vi "create SimpleCredit.vi"(4 "Interest Rate Interval (s)":u32, 5 "Credit Limit Interval (s)":u32, 6 "Interest Rate":dbl, 7 "Credit Limit":dbl, 8 "error in (no error)":errorcluster, 9 "Initial Balance":dbl, 10 "Account Number":string, 11 "SimpleCredit in":refnum<class "SimpleCredit.lvclass">) -> (0 "error out":errorcluster, 3 "SimpleCredit out":refnum<class "SimpleCredit.lvclass">)   [LabVIEW 2020, in "SimpleCredit.lvclass"]
uses:
  SimpleCredit.lvclass
  C:/projects/budget_LabVIEW/Main Codeline/Software/Code/shared/AAccount/AAccount.lvclass
  C:/projects/budget_LabVIEW/Main Codeline/Software/Code/shared/ACreditAccount/ACreditAccount.lvclass
  C:/projects/budget_LabVIEW/Main Codeline/Software/Code/shared/AInterestAccount/AInterestAccount.lvclass
  SimpleCredit.lvclass/SimpleCredit.ctl
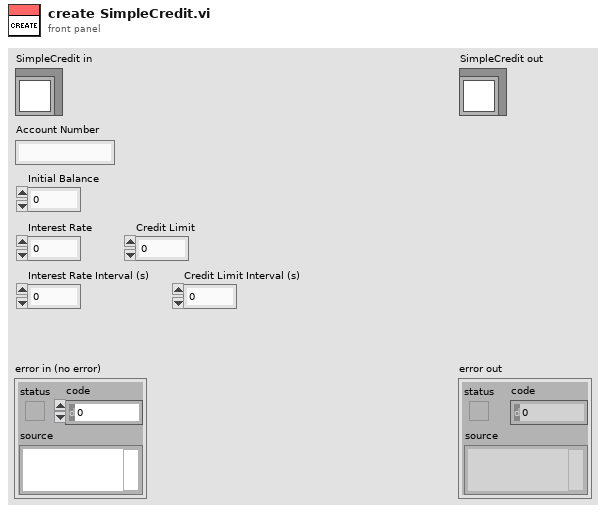
[diagram p1: front panel]
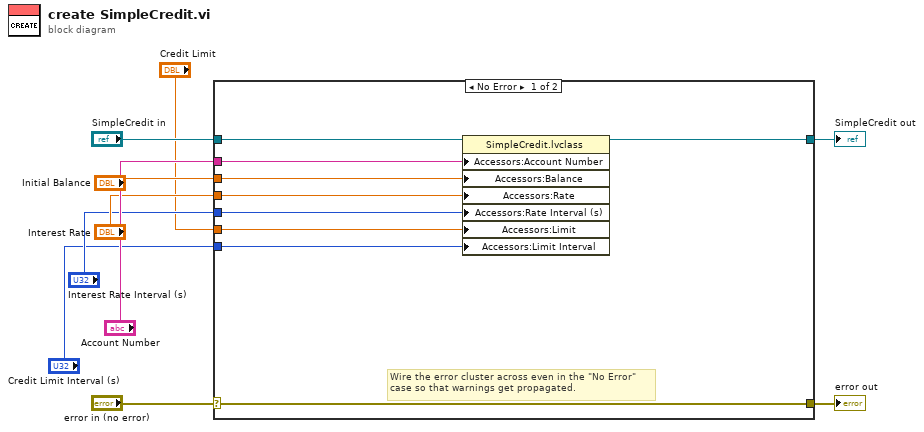
[diagram p0: block diagram]
diagram:
  n1 = case shown="No Error" "error in (no error)" {
    selector: "error in (no error)" -> [w18 w21]
    tunnel: [w18 w21] -> w9
    tunnel: [w17 w20] -> w7
    tunnel: "SimpleCredit in" -> [w19 w20]
    tunnel: "Account Number" -> [w16 _]
    tunnel: "Initial Balance" -> [w15 _]
    tunnel: "Interest Rate" -> [w14 _]
    tunnel: "Interest Rate Interval (s)" -> [w13 _]
    tunnel: "Credit Limit" -> [w12 _]
    tunnel: "Credit Limit Interval (s)" -> [w11 _]
    frame No Error {
      # "Wire the error cluster across even in the \"No Error\"\ncase so that warnings get propagated."
      n2 = property class="SimpleCredit.lvclass"(reference=w19, "Accessors:Account Number"=w16, "Accessors:Balance"=w15, "Accessors:Rate"=w14, "Accessors:Rate Interval (s)"=w13, "Accessors:Limit"=w12, "Accessors:Limit Interval"=w11) -> (reference out=w17:refnum<class "SimpleCredit.lvclass">)  [unwired: 1 in, 1 out]
    }
    frame Error {
    }
  }
  "error out" <- w9
  "SimpleCredit out" <- w7
